vi "dfd_Lattice Level Up.vi"(1 "km":dbl format="%.2f", 2 "Bm-1(z)":dbl[](array[numeric]) format="%.2f") -> (0 "Bm(z)":dbl[](array[numeric]) format="%.2f")   [LabVIEW 2017, in "NI_DigFilterLicensed.lvlib"]
uses:
  <vilib>/addons/Digital Filter Design/NI_DigFilterLicensed.lvlib
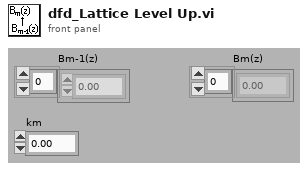
[diagram p1: front panel]
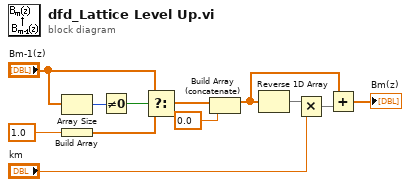
[diagram p0: block diagram]
diagram:
  n1 = Array Size(array="Bm-1(z)") -> (size(s)=w12:i32)
  n2 = Build Array(1.0 ("element")) -> (w8:dbl[])
  n3 = Not Equal To 0?(x=w12) -> (x != 0?=w10:bool)
  n4 = Select(t="Bm-1(z)", s=w10, f=w8) -> (s? t:f=w7:dbl[])
  n5 = Build Array (concatenate)(w7, 0.0) -> (w5:dbl[])
  n6 = Reverse 1D Array(array=w5) -> (reversed array=w4:dbl[])
  n7 = Multiply(x=w4, y="km") -> (x*y=w2:dbl[])
  n8 = Add(x=w5, y=w2) -> (x+y=→"Bm(z)":dbl[])
